vi "Send Current.vi"(8 "error in (no error)":errorcluster, 11 "36234A in":refnum<class "36234A.lvclass">) -> (0 "error out":errorcluster, 3 "36234A out":refnum<class "36234A.lvclass">)   [LabVIEW 2019, in "36234A.lvlib" / "36234A.lvclass"]
uses:
  Library/36234A.lvclass
  C:/Users/Public/Documents/Development/builds/Instruments/PowerSupply.lvlibp/Library/PowerSupply.lvclass
  Library/36234A.lvclass/36234A.ctl
  builds/Instruments/PowerSupply.lvlibp/Accessors/Read Active Channel.vi
  <instrlib>/Keysight E36000 Series/Keysight E36000 Series.lvlib
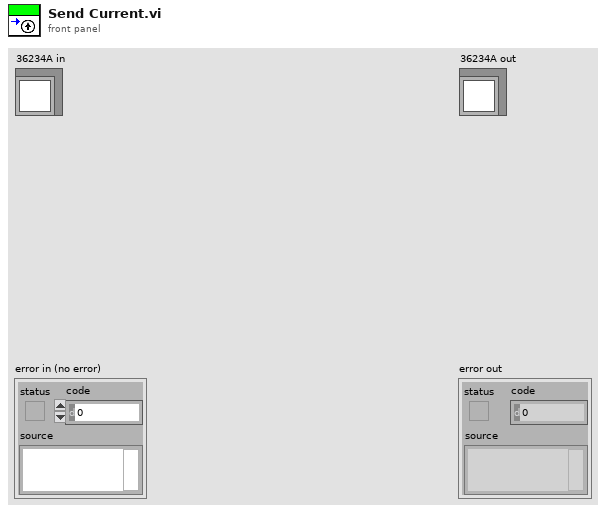
[diagram p1: front panel]
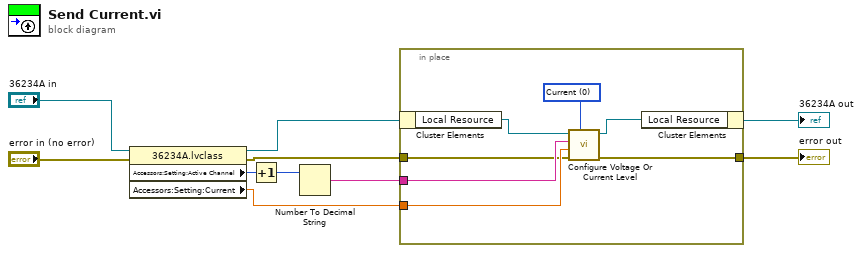
[diagram p0: block diagram]
diagram:
  n1 = property class="36234A.lvclass"(reference="36234A in", error in="error in (no error)") -> (reference out=w7:refnum<class "36234A.lvclass">, error out=w2:errorcluster, "Accessors:Setting:Active Channel"=w10:u32, "Accessors:Setting:Current"=w3:dbl)
  n2 = Increment(x=w10) -> (x+1=w9:u32)
  n3 = Number To Decimal String(number=w9) -> (decimal integer string=w4:string)  [unwired: 1 in]
  n4 = in-place {
    in-place-border: w4 -> [w14]
    in-place-border: w3 -> [w13]
    in-place-border: w2 -> [w12]
    in-place-border: [w11] -> w1
    w15 = 0 items=["Current", "Voltage"] ("Function (0 : Current)")
    n5 = in-place-cluster #1(w7) -> ("Local Resource"=w17:refnum<visa-resource-name>)
    n6 = call <instrlib>:"Configure Voltage Or Current Level.vi"("Function (0 : Current)"=w15, "error in (no error)"=w12, "Voltage Or Current Level (1)"=w13, "Channel (1)"=w14, "VISA resource name"=w17) -> ("error out"=w11:errorcluster, "VISA resource name out"=w16:refnum<visa-resource-name>)  [unwired: 5 in]
    n7 = in-place-cluster #1("Local Resource"=w16) -> (→"36234A out":refnum<class "36234A.lvclass">)
  }
  "error out" <- w1
